vi "Template_Driven_Case.vi"   [LabVIEW 2018]
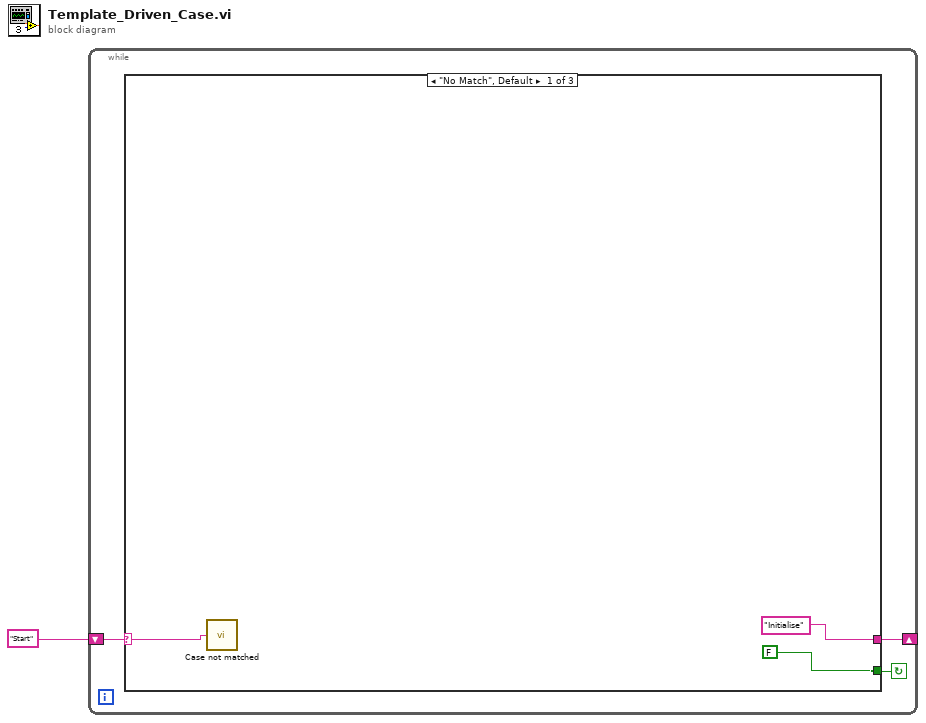
[diagram p0: block diagram]
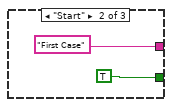
[diagram p2: hidden frame]
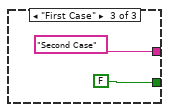
[diagram p3: hidden frame]
diagram:
  n1 = while {
    shift-left: "Start" -> [w2]
    shift-right: [w3] -> _
    stop <- w4 continue-if-true
    n2 = case shown="\"No Match\", Default" w2 {
      selector: w2 -> [w5 _ _]
      tunnel: [FALSE TRUE FALSE] -> w4
      tunnel: ["Initialise" "First Case" "Second Case"] -> w3
      frame "No Match", Default {
        n3 = call "Case not matched.vi"("Case Name not Matched"=w5) -> ()
      }
      frame "Start" {
      }
      frame "First Case" {
      }
    }
  }
